vi "PSU Action Status (Read).vi"(6 "ISOBUS address":T3=-1 caption="ISOBUS address (-1)", 8 "error in":errorcluster, 11 "Mercury Reference In":T4) -> (0 "error out":errorcluster, 2 "PSU Act Stat":T1 caption="PSU Action Status", 3 "Mercury Reference Out":T4, 4 "Valid?":T2)   [LabVIEW 2014, in "Mercury iXX.lvlib" / "Magnet.lvlib"]
doc: "Acquire the most recent PSU action status signal."
uses:
  Magnet.lvlib
  Controls/Mercury Reference.ctl
  Controls/Comms Transport Layer.ctl
  Private/Controls/Query Dynamic Reference.ctl
  Controls/ISOBus Address.ctl
  Controls/Is Valid LED.ctl
  Controls/PSU Actions.ctl
  Private/Controls/Command Verbs.ctl
  Mercury iXX.lvlib
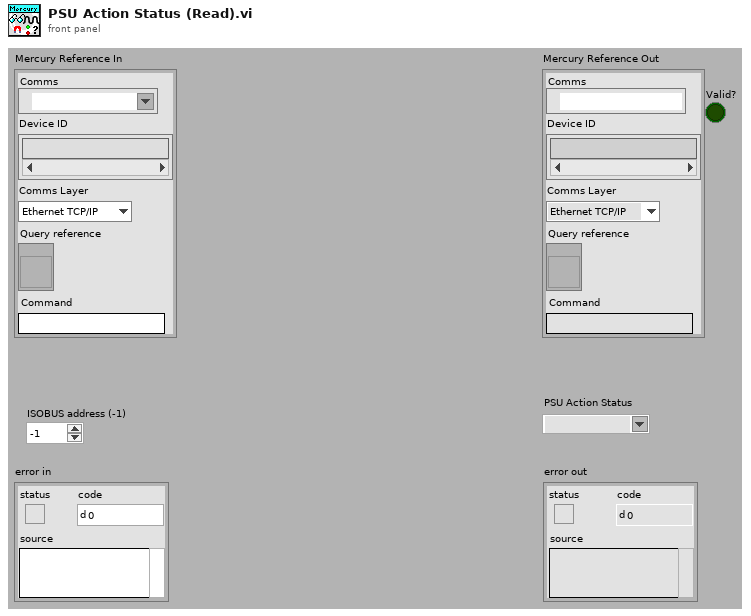
[diagram p1: front panel]
types:
  T1 = typedef "Mercury iXX.lvlib/Magnet.lvlib/PSU Actions.ctl" = string
  T2 = typedef "Mercury iXX.lvlib/Is Valid LED.ctl" = bool
  T3 = typedef "Mercury iXX.lvlib/ISOBus Address.ctl" = i32
  T4 = typedef "Mercury iXX.lvlib/Mercury Reference.ctl" = cluster{"Comms":refnum<visa-resource-name>, "Device ID":string[], "Comms Layer":T5, "Command":string, "Query reference":T6}
  T5 = typedef "Mercury iXX.lvlib/Comms Transport Layer.ctl" = enum16{"Ethernet TCP/IP", "USB", "ISOBus - RS-232", "GPIB"}
  T6 = typedef "Mercury iXX.lvlib/Query Dynamic Reference.ctl" = refnum<vi>
  T7 = typedef "Mercury iXX.lvlib/Command Verbs.ctl" = string
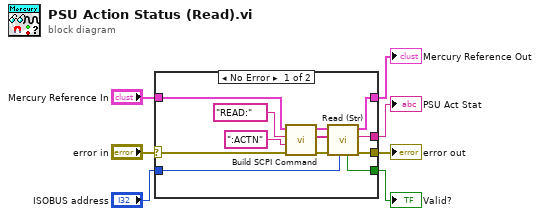
[diagram p0: block diagram]
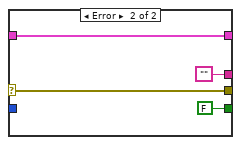
[diagram p2: hidden frame]
diagram:
  n1 = case shown="No Error" "error in" {
    selector: "error in" -> [w8 w22]
    tunnel: [w19 w23] -> w7
    tunnel: [w18 w22] -> w6
    tunnel: [w17 T2 FALSE ("Valid?")] -> w5
    tunnel: "ISOBUS address" -> [w16 _]
    tunnel: [w15 ""] -> w3
    tunnel: "Mercury Reference In" -> [w12 w23]
    frame No Error {
      n2 = call "Build SCPI Command.vi"("error in"=w8, "Noun(s)"=":ACTN" ("Command"), "Verb"=T7 "READ:", "Mercury Reference In"=w12) -> ("error out"=w10:errorcluster, "SCPI Message(s)"=w9:string[], "Mercury Reference Out"=w11:T4)  [unwired: 5 out]
      n3 = call "Read (Str).vi"("ISOBUS address"=w16, "error in"=w10, "SCPI Message(s)"=w9, "Mercury Reference In"=w11) -> ("error out"=w18:errorcluster, "Response"=w15:string, "Mercury Reference Out"=w19:T4, "Valid?"=w17:T2)  [unwired: 4 out]
    }
    frame Error {
    }
  }
  "Mercury Reference Out" <- w7
  "error out" <- w6
  "Valid?" <- w5
  "PSU Act Stat" <- w3
